vi "camToRobotTranslate.vi"(8 "camOffset":T1, 10 "camDistToGoal":dbl, 11 "camAngleToGoal":dbl) -> (0 "robotDistToGoal":dbl, 3 "robotAngleToGoal":dbl)   [LabVIEW 2016]
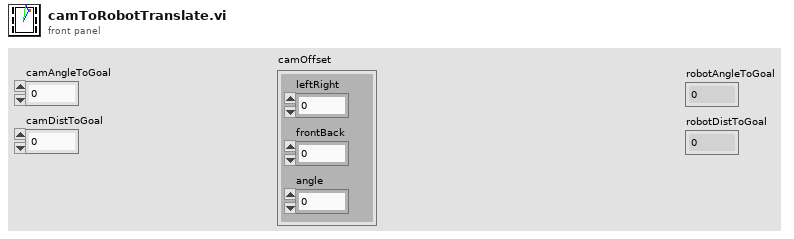
[diagram p1: front panel]
types:
  T1 = cluster{"leftRight":dbl, "frontBack":dbl, "angle":dbl}
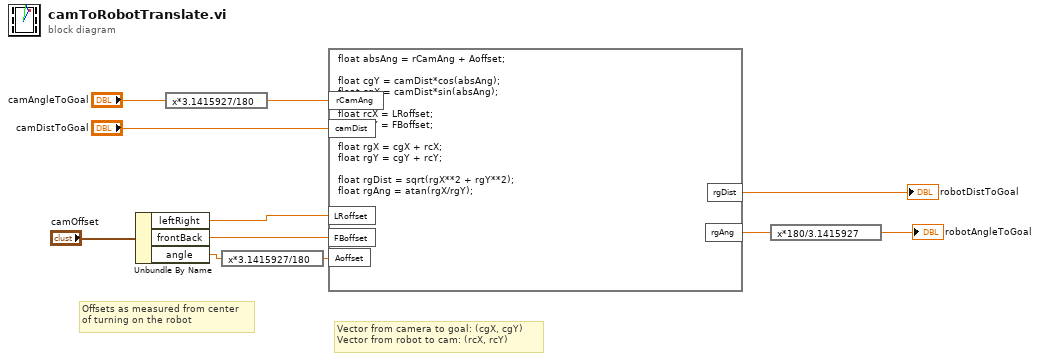
[diagram p0: block diagram]
diagram:
  # "Offsets as measured from center\nof turning on the robot"
  # "Vector from camera to goal: (cgX, cgY)\nVector from robot to cam: (rcX, rcY)"
  n1 = Unbundle By Name("camOffset") -> ("leftRight"=w7:dbl, "frontBack"=w6:dbl, "angle"=w5:dbl)
  n2 = expression code="x*3.1415927/180"("camAngleToGoal") -> (w9:dbl)
  n3 = expression code="x*3.1415927/180"(w5) -> (w4:dbl)
  n4 = formula code="float absAng = rCamAng + Aoffset;\n\nfloat cgY = camDist*cos(absAng);\nfloat cgX = camDist*sin(absAng);\n\nfloat rcX = LRoffset;\nfloat rcY = FBoffset;\n\nfloat rgX = cgX + rcX;\nfloat rgY = cgY + rcY;\n\nfloat rgDist = sqrt(rgX**2 + rgY**2);\nfloat rgAng = atan(rgX/rgY);"("rCamAng"=w9, "camDist"="camDistToGoal", "LRoffset"=w7, "FBoffset"=w6, "Aoffset"=w4) -> ("rgDist"=→"robotDistToGoal":dbl, "rgAng"=w3:dbl)
  n5 = expression code="x*180/3.1415927"(w3) -> (→"robotAngleToGoal":dbl)
